vi "Idling.vi"(9 "Exit Ref":refnum<vi>, 10 "Start Ref":refnum<vi>, 11 "Go to Idle?":T1) -> (1 "Exit":T1, 2 "Make Measurement":T1, 3 "Return to Idling":T1)   [LabVIEW 2017]
uses:
  <extravilib>/ChannelInstances/Messenger-bool/))Channel.ctl
  <extravilib>/ChannelInstances/Messenger-bool/Read With Abort.vi
  <extravilib>/ChannelInstances/Messenger-bool/Write With Abort.vi
  <resource>/Channels/Messenger/Read With Abort.vi
  <vilib>/ChannelSupport/Channel Message/Read ID.vi
  <resource>/Channels/Messenger/Write With Abort.vi
  <extravilib>/ChannelInstances/Messenger-bool/Wrapper.lvclass
  C:/Program Files (x86)/National Instruments/LabVIEW 2017/vi.lib/ChannelSupport/Channel Message/Channel Message.lvclass
  <resource>/Channels/Messenger/Endpoint.vi
  <extravilib>/ChannelInstances/Messenger-bool/Unwrap.vi
  <extravilib>/ChannelInstances/Messenger-bool/Wrap.vi
  <extravilib>/ChannelInstances/Messenger-bool.lvlib
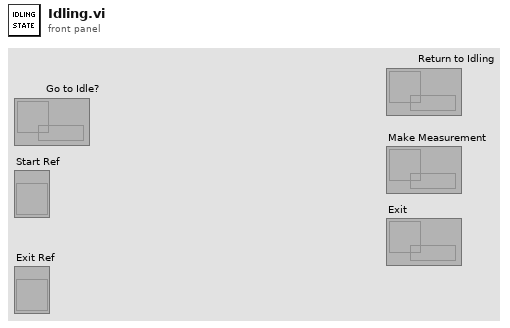
[diagram p1: front panel]
types:
  T1 = typedef "Messenger-bool.lvlib/))Channel.ctl" = refnum<queue>
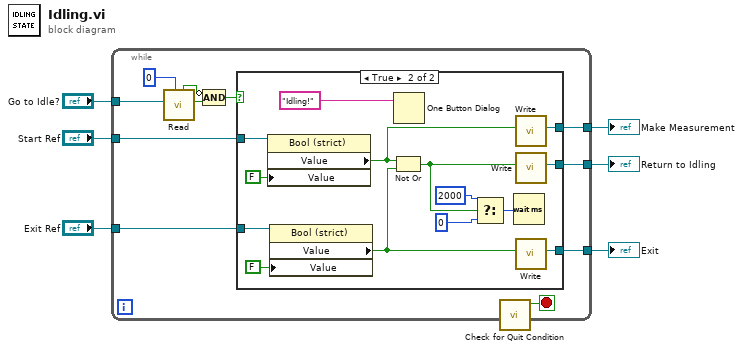
[diagram p0: block diagram]
diagram:
  n1 = while {
    tunnel: "Go to Idle?" -> [w17]
    tunnel: [w15] -> w5
    tunnel: [w14] -> w4
    tunnel: [w13] -> w3
    tunnel: "Start Ref" -> [w8]
    tunnel: "Exit Ref" -> [w7]
    stop <- w9 stop-if-true
    n2 = call <extravilib>:"Read.vi"("timeout in ms (-1)"=0, "channel"=w17) -> ("element"=w16:bool, "timedout?"=w11:bool)  [unwired: 6 in, 2 out]
    n3 = Compound Arithmetic op=AND(invert w11, w16) -> (w12:bool)
    n4 = case shown="True" w12 {
      tunnel: [_ w30] -> w15
      tunnel: [_ w29] -> w14
      tunnel: [_ w28] -> w13
      tunnel: w8 -> [_ w23]
      tunnel: w7 -> [_ w21]
      frame False {
      }
      frame True {
        n5 = property class="Bool (strict)"(reference=w23, "Value"=FALSE) -> ("Value"=w20:bool)  [unwired: 1 in, 2 out]
        n6 = property class="Bool (strict)"(reference=w21, "Value"=FALSE) -> ("Value"=w22:bool)  [unwired: 1 in, 2 out]
        n7 = Not Or(1:w22, 2:w20) -> (0:w27:bool)
        n8 = One Button Dialog(message="Idling!") -> ()  [unwired: 1 in, 1 out]
        n9 = Select(t=u32 2000, s=w27, f=u32 0) -> (s? t:f=w24:u32)
        n10 = Wait (ms)(milliseconds to wait=w24) -> ()  [unwired: 1 out]
        n11 = call <extravilib>:"Write.vi"("element"=w20) -> ("channel"=w29:T1)  [unwired: 8 in, 2 out]
        n12 = call <extravilib>:"Write.vi"("element"=w27) -> ("channel"=w30:T1)  [unwired: 8 in, 2 out]
        n13 = call <extravilib>:"Write.vi"("element"=w22) -> ("channel"=w28:T1)  [unwired: 8 in, 2 out]
      }
    }
    n14 = call "Check for Quit Condition.vi"() -> ("Quit?"=w9:bool)  [unwired: 11 in]
  }
  "Return to Idling" <- w5
  "Make Measurement" <- w4
  "Exit" <- w3
